vi "TimeoutWrite buffers BjusticeData.vi"(6 "data rate (hz)":dbl format="%#_13g", 7 "previous timestamp":dbl, 11 "Map":map{string, T1}(c390)) -> (5 "current timestamp":dbl)   [LabVIEW 2021, in "RocketPlotDemo.lvlib"]
uses:
  RocketPlotDemo.lvlib
  <userlib>/bjustice/Ring Buffer for Time Series Data Strict Accessor/SubVIs/RingBufferHandle.ctl
  <userlib>/bjustice/Ring Buffer for Time Series Data/SubVIs/DVR data.ctl
  <userlib>/bjustice/Ring Buffer for Time Series Data Strict Accessor/SubVIs/DataType.ctl
  <userlib>/bjustice/Ring Buffer for Time Series Data Strict Accessor/SubVIs/Endianess.ctl
  5b9cd612-4a81-4300-8a75-0b992cbc4093.vi
  1f7b7afb-48a8-4668-891f-f005d6994698.vi
  36cc8d9c-9779-4c8a-a9b9-37b0beffe98c.vi
  <userlib>/bjustice/Ring Buffer for Time Series Data Strict Accessor/Unix time epoch/Unix_Epoch_in_Labview.vi
  <userlib>/bjustice/Ring Buffer for Time Series Data/API Poly.vi
  <userlib>/bjustice/Ring Buffer for Time Series Data/API/Write Array.vi
  36cc8d9c-9779-4c8a-a9b9-37b0beffe98c.vi/f2df9050-0eef-46c6-aff6-3ce3a8893ea5.vi
  <userlib>/bjustice/Ring Buffer for Time Series Data/SubVIs/Split Values Array.vi
  <userlib>/bjustice/Ring Buffer for Time Series Data/SubVIs/Replace Values Array Multiple Timestamps.vi
  36cc8d9c-9779-4c8a-a9b9-37b0beffe98c.vi/f2df9050-0eef-46c6-aff6-3ce3a8893ea5.vi/63c583a5-c20f-4aba-9c90-661423dee4c4.vi
  36cc8d9c-9779-4c8a-a9b9-37b0beffe98c.vi/f2df9050-0eef-46c6-aff6-3ce3a8893ea5.vi/52385341-3d9c-45d2-aff5-e082a4793eb1.vi
  36cc8d9c-9779-4c8a-a9b9-37b0beffe98c.vi/f2df9050-0eef-46c6-aff6-3ce3a8893ea5.vi/37f29efa-f142-46b1-a185-f0098a95fbb6.vi
  36cc8d9c-9779-4c8a-a9b9-37b0beffe98c.vi/f2df9050-0eef-46c6-aff6-3ce3a8893ea5.vi/84b3d231-9afe-4b6e-afae-e0be43a31e4e.vi
  36cc8d9c-9779-4c8a-a9b9-37b0beffe98c.vi/f2df9050-0eef-46c6-aff6-3ce3a8893ea5.vi/c726271c-fc36-4bb7-8553-8945ec40c1cd.vi
  36cc8d9c-9779-4c8a-a9b9-37b0beffe98c.vi/f2df9050-0eef-46c6-aff6-3ce3a8893ea5.vi/a7b1d944-dc88-46f5-9d3e-305d46bbe1f6.vi
  36cc8d9c-9779-4c8a-a9b9-37b0beffe98c.vi/f2df9050-0eef-46c6-aff6-3ce3a8893ea5.vi/8abc4a6e-a1d2-4e85-879b-517e0ab55733.vi
  36cc8d9c-9779-4c8a-a9b9-37b0beffe98c.vi/f2df9050-0eef-46c6-aff6-3ce3a8893ea5.vi/bd347357-b475-4a03-9ac5-3b85ef11aecc.vi
  36cc8d9c-9779-4c8a-a9b9-37b0beffe98c.vi/f2df9050-0eef-46c6-aff6-3ce3a8893ea5.vi/391b36e9-a702-45e4-9499-3914f8833a58.vi
  36cc8d9c-9779-4c8a-a9b9-37b0beffe98c.vi/f2df9050-0eef-46c6-aff6-3ce3a8893ea5.vi/44155b33-c915-49ce-9e44-a66693aa70dd.vi
  36cc8d9c-9779-4c8a-a9b9-37b0beffe98c.vi/f2df9050-0eef-46c6-aff6-3ce3a8893ea5.vi/36977d53-dbe0-4dbc-b2ac-3dea4345b868.vi
  <userlib>/bjustice/Ring Buffer for Time Series Data/SubVIs/Enforce array size multiple timestamps.vi
  <vilib>/Utility/error.llb/Error Cluster From Error Code.vi
  <userlib>/bjustice/Ring Buffer for Time Series Data Strict Accessor/Ring Buffer Strict Accessor.lvlib
  <userlib>/bjustice/Ring Buffer for Time Series Data/Ring Buffer Time Series Data.lvlib
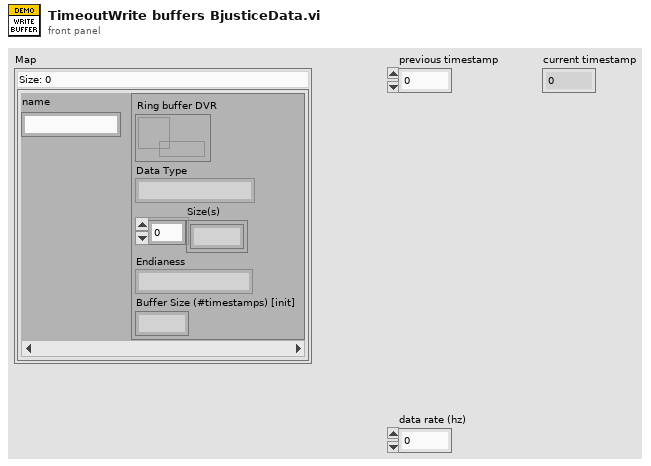
[diagram p1: front panel]
types:
  T1 = typedef "Ring Buffer Strict Accessor.lvlib/RingBufferHandle.ctl" = cluster{"Ring buffer DVR":refnum<data-value>, "Data Type":T2, "Size(s)":i32[], "Endianess":T3, "Buffer Size (#timestamps) [init]":i32}
  T2 = typedef "Ring Buffer Strict Accessor.lvlib/DataType.ctl" = enum16{"uint8", "uint16", "uint32", "uint64", "int8", "int16", "int32", "int64", "float", "double", "extended"}
  T3 = typedef "Ring Buffer Strict Accessor.lvlib/Endianess.ctl" = enum16{"big-endian", "little-endian"}
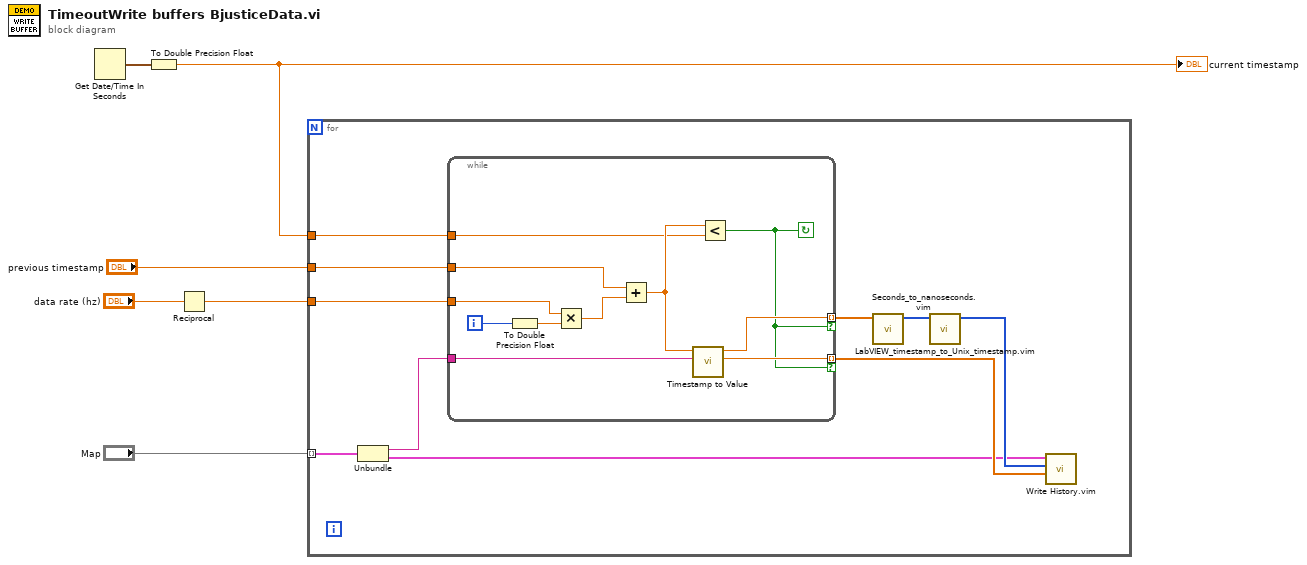
[diagram p0: block diagram]
diagram:
  n1 = Get Date/Time In Seconds() -> (seconds since 1Jan1904=w6:timestamp)
  n2 = To Double Precision Float(number=w6) -> (double precision float=w1:dbl)
  "current timestamp" <- w1
  n3 = Reciprocal(x="data rate (hz)") -> (1/x=w3:dbl)
  n4 = for {
    tunnel: "Map" -> [w12] mode=indexing
    tunnel: w3 -> [w10]
    tunnel: "previous timestamp" -> [w9]
    tunnel: w1 -> [w8]
    n5 = Unbundle(w12) -> ("name"=w11:string, "Ring Buffer"=w7:T1)
    n6 = while {
      tunnel: w11 -> [w27]
      tunnel: [w26] -> w16 mode=indexing if=w17
      tunnel: [w25] -> w13 mode=indexing if=w17
      tunnel: w10 -> [w23]
      tunnel: w9 -> [w21]
      tunnel: w8 -> [w18]
      i -> [w20]
      stop <- w17 continue-if-true
      n7 = To Double Precision Float(number=w20) -> (double precision float=w24:dbl)
      n8 = Multiply(x=w23, y=w24) -> (x*y=w22:dbl)
      n9 = Add(x=w21, y=w22) -> (x+y=w19:dbl)
      n10 = call "Timestamp to Value.vi"("name"=w27, "timestamp"=w19) -> ("value"=w25:dbl, "timestamp (dup)"=w26:dbl)  [unwired: 8 in]
      n11 = Less?(x=w19, y=w18) -> (x < y?=w17:bool)
    }
    n12 = call "Seconds_to_nanoseconds.vim"("timestamp (seconds)"=w16) -> ("timestamp (nanoseconds)"=w15:u64[])  [unwired: 10 in]
    n13 = call "LabVIEW_timestamp_to_Unix_timestamp.vim"("LabVIEW timestamp (nanoseconds)"=w15) -> ("Unix timestamp (nanoseconds)"=w14:u64[])  [unwired: 10 in]
    n14 = call "Write History.vim"("LV DataType"=w13, "Timestamps"=w14, "Ring Buffer"=w7) -> ()  [unwired: 7 in, 2 out]
  }
